vi "UDP Available Test.vi"() -> ()   [LabVIEW 2014, in "ESP8266 WiFi Wrapper.lvlib"]
uses:
  ESP8266 WiFi Wrapper.lvlib
panel:
  out "Available?":u8
  out "Error Out":errorcluster
  in  "Error In":errorcluster
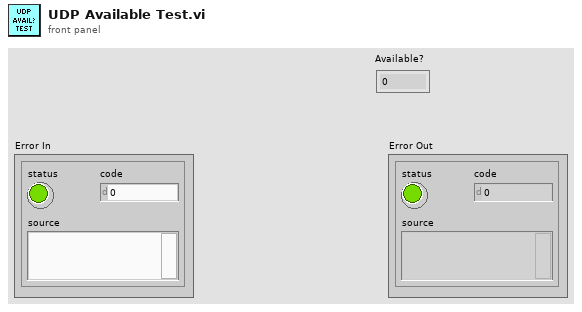
[diagram p1: front panel]
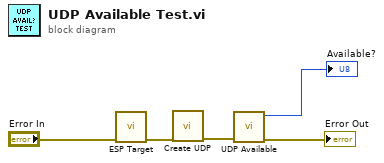
[diagram p0: block diagram]
diagram:
  n1 = call "ESP Target.vi"("Error In"="Error In") -> ("Error Out"=w2:errorcluster)  [unwired: 10 in]
  n2 = call "Create UDP.vi"("Error In"=w2) -> ("Error Out"=w1:errorcluster)  [unwired: 10 in]
  n3 = call "UDP Available.vi"("Error In"=w1) -> ("Error Out"=→"Error Out":errorcluster, "Available?"=→"Available?":u8)  [unwired: 9 in]
